vi "双路Preview Start.vi"(8 "error in":errorcluster, 10 "preview path":u8) -> (0 "error out":errorcluster, 2 "return":i32)   [LabVIEW 2016]
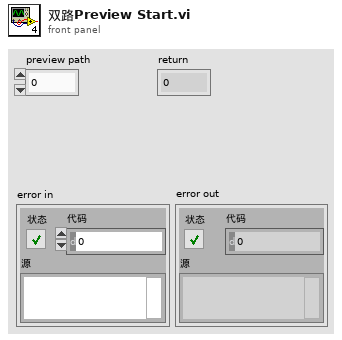
[diagram p1: front panel]
types:
  T1 = cluster{"byCmdType":u8, "bySubCmd":u8, "byPara":u8, "byAddr_h":u8, "byAddr_l":u8, "byAddr_ll":u8, "byLen_h":u8, "byLen_l":u8}
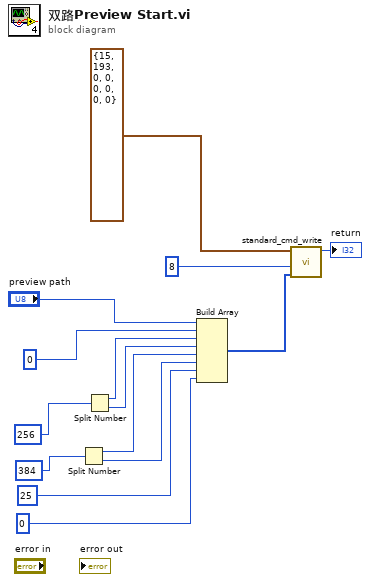
[diagram p0: block diagram]
diagram:
  n1 = Split Number(x=u16 384) -> (hi(x)=w7:u8, lo(x)=w6:u8)
  n2 = Split Number(x=u16 256) -> (hi(x)=w9:u8, lo(x)=w8:u8)
  n3 = Build Array("preview path", u8 0, w9, w8, w7, w6, u8 25, u8 0) -> (w3:u8[])
  n4 = call "standard_cmd_write.vi"("data"=w3, "dwLen"=u32 8, "cmd_std_header_t"=T1 {"byCmdType"=15, "bySubCmd"=193, "byPara"=0, "byAddr_h"=0, "byAddr_l"=0, "byAddr_ll"=0, "byLen_h"=0, "byLen_l"=0}) -> ("return"=→"return":i32)  [unwired: 8 in]
